vi "SFP_WMF_Excel_Message.vi"() -> (3 "message out":string)   [LabVIEW 2020]
panel:
  in  "message":string="Failed to save this VI.\n\nYour VI contains the Write To Measurement File Express VI, which does not support the Microsoft Excel file format in the specified version of LabVIEW. You must configure this Express VI to use other file formats before saving it for a previous version of LabVIEW."
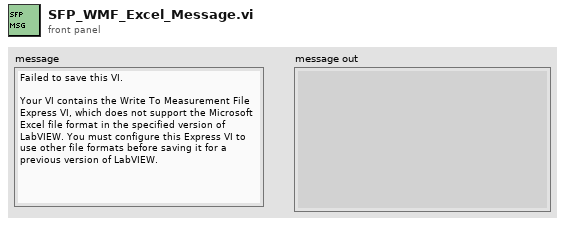
[diagram p1: front panel]
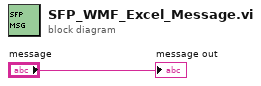
[diagram p0: block diagram]
diagram:
  "message out" <- "message"
